vi "Actor Core.vi"(8 "error in":errorcluster, 11 "Camera Dir Dialog in":refnum<class "Camera Dir Dialog.lvclass">) -> (0 "error out":errorcluster, 3 "Actor out":refnum<class "Actor.lvclass">)   [LabVIEW 2014, in "Camera Dir Dialog.lvlib" / "Camera Dir Dialog.lvclass"]
doc: "(<B>Filename</B>: Actor Framework.lvlib:Actor.lvclass:Actor Core.vi)\n\nReceives messages to the actor, reacts to them, and initiates any error handling that may shut the actor down.\n\nDescendant classes may override this VI to append parallel tasks for the actor to complete while it handles messages. Overrides use the Call Parent Method node."
uses:
  Camera Dir Dialog.lvclass
  <vilib>/ActorFramework/Actor/Actor.lvclass
  Camera Dir Dialog.lvclass/Camera Dir Dialog.ctl
  <vilib>/ActorFramework/Actor/Actor.lvclass/Actor.ctl
  <vilib>/ActorFramework/Message Enqueuer/Message Enqueuer.lvclass/Message Enqueuer.ctl
  Camera Dir Dialog Messages/Write Config Dir Msg/Write Config Dir Msg.lvclass/Write Config Dir Msg.ctl
  Camera Dir Dialog Messages/Write WorkDir Msg/Write WorkDir Msg.lvclass/Write WorkDir Msg.ctl
  Read Config Dir.vi
  Read WorkDir.vi
  <vilib>/ActorFramework/Message Enqueuer/Init from Existing Queue.vi
  <vilib>/ActorFramework/Message Enqueuer/Enqueue.vi
  <vilib>/ActorFramework/Message Priority Queue/Priority Enqueue.vi
  <vilib>/ActorFramework/Message Enqueuer/Message Enqueuer.lvclass
  Camera Dir Dialog Messages/Write Config Dir Msg/Write Config Dir Msg.lvclass
  Camera Dir Dialog Messages/Write WorkDir Msg/Write WorkDir Msg.lvclass
  <vilib>/ActorFramework/Stop Msg/Stop Msg.lvclass
panel:
  in  "Stop Signal":bool=TRUE
  in  "WorkDir":path=path "D:/Test XDisplay images"
  in  "Config Dir":path=path "D:/Test XDisplay images"
  in  "OK Button":bool
  in  "Cancel":bool
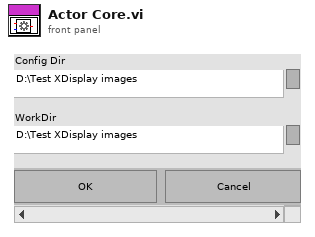
[diagram p1: front panel]
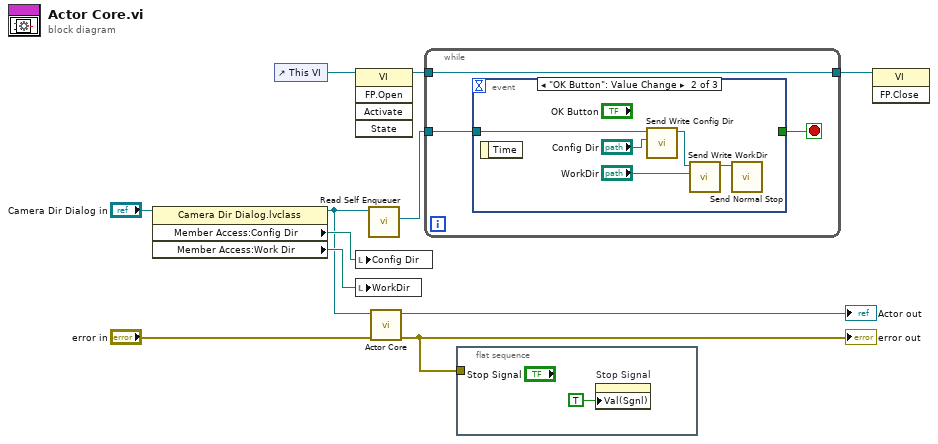
[diagram p0: block diagram]
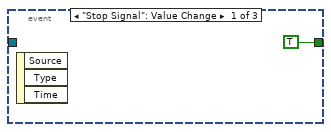
[diagram p2: hidden frame]
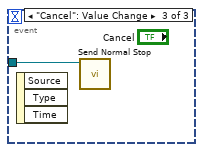
[diagram p3: hidden frame]
diagram:
  n1 = property class="Camera Dir Dialog.lvclass"(reference="Camera Dir Dialog in") -> (reference out=w4:refnum<class "Camera Dir Dialog.lvclass">, "Member Access:Config Dir"=w6:path, "Member Access:Work Dir"=w7:path)  [unwired: 1 in, 1 out]
  n2 = control-ref of="This VI"() -> (w3:refnum<vi>)
  n3 = invoke class="VI" method="FP.Open"(reference=w3) -> (reference out=w2:refnum<vi>)  [unwired: 4 in, 4 out]
  n4 = local write "Config Dir"(w6) -> ()
  n5 = local write "WorkDir"(w7) -> ()
  n6 = call <vilib>:"Read Self Enqueuer.vi"("Actor"=w4) -> ("Self Enqueuer"=w5:refnum<class "Message Enqueuer.lvclass">)  [unwired: 10 in]
  n7 = call-parent "Actor Core.vi"("error in"="error in", "Actor in"=w4) -> ("error out"=w8:errorcluster, "Actor out"=→"Actor out":refnum<class "Actor.lvclass">)  [unwired: 8 in]
  "error out" <- w8
  n8 = while {
    tunnel: w5 -> [w13]
    tunnel: w2 -> [w12]
    tunnel: [w12] -> w1
    stop <- w14 stop-if-true
    n9 = event shown="[1] \"OK Button\": Value Change" {
      selector: _ -> [_ _ _]
      dyn-events: _ -> [_ _ _]
      timeout: _ -> [_ _ _]
      tunnel: [TRUE _ _] -> w14
      tunnel: w13 -> [_ w20 w21]
      event "Stop Signal": Value Change {
        n10 = event-data() -> ()  [unwired: 1 in, 3 out]
      }
      event "OK Button": Value Change {
        n11 = event-data() -> ()  [unwired: 1 in, 1 out]
        n12 = call "Send Write Config Dir.vi"("Config Dir"="Config Dir", "Message Enqueuer"=w20) -> ("Message Enqueuer out"=w19:refnum<class "Message Enqueuer.lvclass">)  [unwired: 8 in, 1 out]
        n13 = call "Send Write WorkDir.vi"("WorkDir"="WorkDir", "Message Enqueuer"=w19) -> ("Message Enqueuer out"=w16:refnum<class "Message Enqueuer.lvclass">)  [unwired: 8 in, 1 out]
        n14 = call <vilib>:"Send Normal Stop.vi"("Message Enqueuer"=w16) -> ()  [unwired: 10 in, 1 out]
      }
      event "Cancel": Value Change {
        n15 = event-data() -> ()  [unwired: 1 in, 3 out]
        n16 = call <vilib>:"Send Normal Stop.vi"("Message Enqueuer"=w21) -> ()  [unwired: 10 in, 1 out]
      }
    }
  }
  n17 = flat-sequence {
    tunnel: w8 -> [_]
    frame #0 {
      n18 = property on="Stop Signal" class="Bool (strict)"("Val(Sgnl)"=TRUE) -> ()  [unwired: 2 in, 2 out]
    }
  }
  n19 = invoke class="VI" method="FP.Close"(reference=w1) -> ()  [unwired: 2 in, 3 out]
